vi "UsrProfiles-Last used name change-Update key.vi"(8 "error in (no error)":errorcluster, 10 "Modified profile name":string) -> (0 "error out":errorcluster)   [LabVIEW 2017]
uses:
  Typedefs/Which path.ctl
  <vilib>/Utility/config.llb/Write Key (String).vi
  <vilib>/Utility/config.llb/NI_LVConfig.lvlib
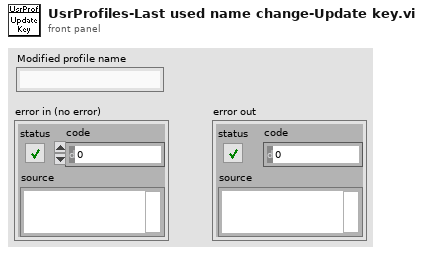
[diagram p1: front panel]
types:
  T1 = typedef "Which path.ctl" = enum16{"Configuration Files", "Calibration Files", "Images", "Setup.ini", "Loaded User profile.ini", "User's-Previous session.ini", "New user profile.ini", "Selected User profile.ini", "User profiles folder", "Power meter scaling.txt", "FOV Cal.ini"}
  T2 = typedef "NI_LVConfig.lvlib/Config Data RefNum.ctl" = refnum<k1>
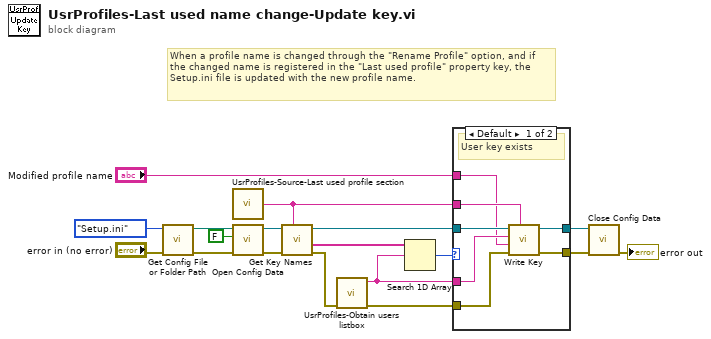
[diagram p0: block diagram]
diagram:
  # "When a profile name is changed through the \"Rename Profile\" option, and if the changed name is registered in the \"Last used profile\" property key, the Setup.ini file is updated with the new profile name."
  n1 = call "Get Config File or Folder Path.vi"("Error In"="error in (no error)", "Which file or folder?"=Which_path."Setup.ini") -> ("Error Out"=w15:errorcluster, "File Path"=w17:path)  [unwired: 7 in, 1 out]
  n2 = call "UsrProfiles-Source-Last used profile section.vi"() -> ("Last Used Profile section name"=w4:string)  [unwired: 1 in]
  n3 = call <vilib>:"Open Config Data.vi"("error in (no error)"=w15, "create file if necessary (T)"=FALSE, "configuration file path"=w17) -> ("error out"=w12:errorcluster, "refnum"=w11:T2)  [unwired: 6 in, 1 out]
  n4 = call <vilib>:"Get Key Names.vi"("section"=w4, "error in (no error)"=w12, "refnum"=w11) -> ("error out"=w3:errorcluster, "key names"=w10:string[], "refnum out"=w7:T2)  [unwired: 5 in, 1 out]
  n5 = call "UsrProfiles-Obtain users listbox.vi"("error in (no error)"=w3) -> ("error out"=w2:errorcluster, "Selected user's name"=w5:string)  [unwired: 7 in, 2 out]
  n6 = Search 1D Array(1D array=w10, element=w5) -> (index of element=w9:i32)  [unwired: 1 in]
  n7 = case shown="Default" w9 {
    tunnel: w2 -> [w23 w27]
    tunnel: [w22 w27] -> w8
    tunnel: w7 -> [w25 w26]
    tunnel: [w24 w26] -> w6
    tunnel: w5 -> [w21 _]
    tunnel: w4 -> [w20 _]
    tunnel: "Modified profile name" -> [w19 _]
    frame Default {
      # "User key exists"
      n8 = call-poly <vilib>:"Write Key.vi"("section"=w20, "error in (no error)"=w23, "value"=w19, "key"=w21, "refnum"=w25) -> ("error out"=w22:errorcluster, "refnum out"=w24:T2)  [unwired: 4 in, 1 out]
    }
    frame -1 {
    }
  }
  n9 = call <vilib>:"Close Config Data.vi"("error in (no error)"=w8, "refnum"=w6) -> ("error out"=→"error out":errorcluster)  [unwired: 8 in, 1 out]
